vi "Transformation Matrix to 3D Model View Matrix.vi"(1 "Transformation Matrix":T1) -> (0 "3D-Control Model Matrix":T1)   [LabVIEW 2020, in "ar.lvlib"]
uses:
  ar.lvlib
  <vilib>/Analysis/Matrix/Datatypes/RealMatrix.ctl
  <vilib>/Analysis/baseanly.llb/Real A x B.vi
  <vilib>/Analysis/NI_AALBase.lvlib
  <vilib>/Analysis/Matrix/NI_Matrix.lvlib
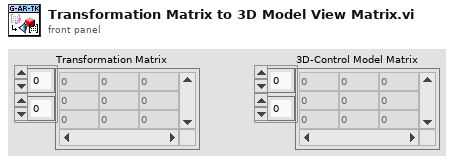
[diagram p1: front panel]
types:
  T1 = typedef "NI_Matrix.lvlib/RealMatrix.ctl" = dbl[][]
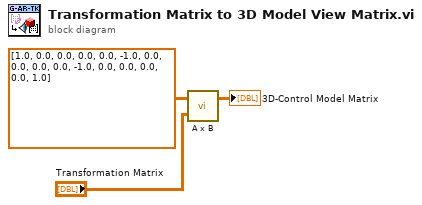
[diagram p0: block diagram]
diagram:
  n1 = call-poly <vilib>:"A x B.vi"("B"="Transformation Matrix", "A"=dbl[][] [[1.0, 0.0, 0.0, 0.0], [0.0, -1.0, 0.0, 0.0], [0.0, 0.0, -1.0, 0.0], [0.0, 0.0, 0.0, 1.0]]) -> ("A x B"=→"3D-Control Model Matrix":T1)  [unwired: 1 out]
